vi "x_var.vi"() -> ()   [LabVIEW 2022 SP3]
panel:
  in  "X":dbl
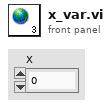
[diagram p1: front panel]
diagram:
